vi "Start Async.vi"(8 "error in (no error)":errorcluster, 11 "gRPC Server in":refnum<class "TestService.lvclass">) -> (0 "error out":errorcluster, 3 "gRPC Server out":refnum<class "TestService.lvclass">)   [LabVIEW 2021, in "test_service_server.lvlib" / "TestService.lvclass"]
uses:
  TestService.lvclass
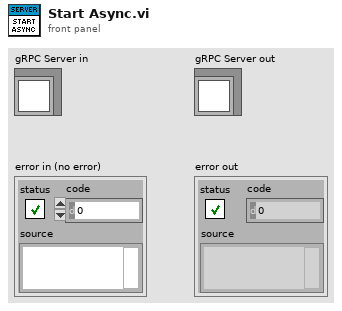
[diagram p1: front panel]
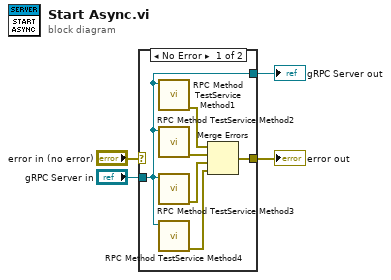
[diagram p0: block diagram]
diagram:
  n1 = case shown="No Error" "error in (no error)" {
    selector: "error in (no error)" -> [_ w12]
    tunnel: [w10 w12] -> w3
    tunnel: [w9 w11] -> w1
    tunnel: "gRPC Server in" -> [w9 w11]
    frame No Error {
      n2 = call "RPC Method TestService Method1.vi"("OOP Server in"=w9) -> ("error out"=w8:errorcluster)  [unwired: 9 in, 1 out]
      n3 = call "RPC Method TestService Method2.vi"("OOP Server in"=w9) -> ("error out"=w7:errorcluster)  [unwired: 9 in, 1 out]
      n4 = call "RPC Method TestService Method3.vi"("OOP Server in"=w9) -> ("error out"=w6:errorcluster)  [unwired: 9 in, 1 out]
      n5 = call "RPC Method TestService Method4.vi"("OOP Server in"=w9) -> ("error out"=w5:errorcluster)  [unwired: 9 in, 1 out]
      n6 = Merge Errors(w8, w7, w6, w5) -> (w10:errorcluster)
    }
    frame Error {
    }
  }
  "error out" <- w3
  "gRPC Server out" <- w1
